vi "Write Homing.vi"(8 "error in (no error)":errorcluster, 10 "Homing":variant, 11 "Filter Wheel in":refnum<class "Filter Wheel.lvclass">) -> (0 "error out":errorcluster, 3 "Filter Wheel out":refnum<class "Filter Wheel.lvclass">)   [LabVIEW 2024, in "Filter Wheel.lvclass"]
uses:
  Filter Wheel.lvclass
  Filter Wheel Arduino Control/Filter Wheel Arduino Homing cluster.ctl
  Filter Wheel.lvclass/Filter Wheel.ctl
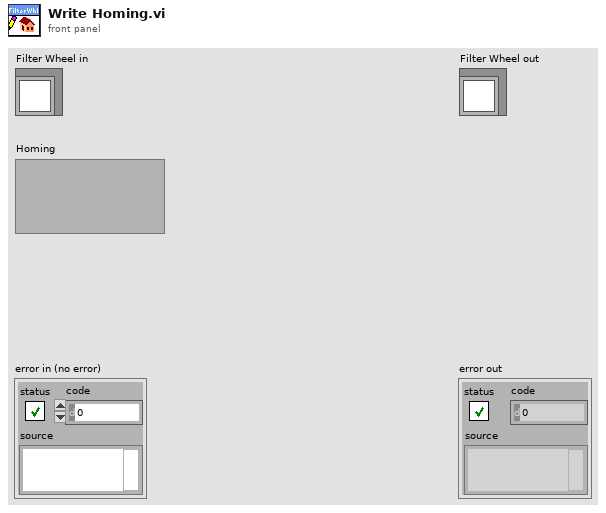
[diagram p1: front panel]
types:
  T1 = typedef "Filter Wheel Arduino Homing cluster.ctl" = cluster{"Direction (F: CW)":bool, "Speed":i32, "Accel":i32, "Min Distance":i32, "Short Leg":i32, "Error Cnts":i32}
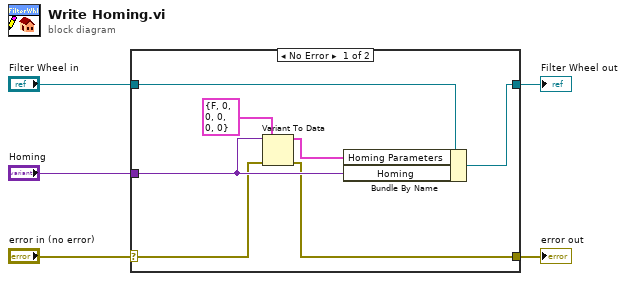
[diagram p0: block diagram]
diagram:
  n1 = case shown="No Error" "error in (no error)" {
    selector: "error in (no error)" -> [w7 w13]
    tunnel: [w6 w13] -> w4
    tunnel: [w11 w14] -> w2
    tunnel: "Filter Wheel in" -> [w12 w14]
    tunnel: "Homing" -> [w9 _]
    frame No Error {
      n2 = Variant To Data(error in=w7, type=T1 {"Direction (F: CW)"=FALSE, "Speed"=0, "Accel"=0, "Min Distance"=0, "Short Leg"=0, "Error Cnts"=0} ("Homing Parameters"), Variant=w9) -> (data=w8:T1, error out=w6:errorcluster)
      n3 = Bundle By Name(cluster=w12, "Homing Parameters"=w8, "Homing"=w9) -> (w11:refnum<class "Filter Wheel.lvclass">)
    }
    frame Error {
    }
  }
  "error out" <- w4
  "Filter Wheel out" <- w2
